vi "_FG_save_hth_v6.vi"(0 "Énum":T1, 1 "array 1":dbl[](array[numeric]), 3 "array 2":dbl[](array[numeric]), 4 "array 3":dbl[](array[numeric]), 5 "error in":errorcluster, 6 "antet_files":string, 7 "write to raw data ?":bool, 8 "add EOL at end ?":bool, 9 "text before data":string, 11 "text":string, 12 "cluster of arrays":cluster{dbl, dbl}[](array[cluster]), 13 "format":string="%12.9g") -> (19 "error out":errorcluster)   [LabVIEW 2017]
uses:
  controls/save_data_hth_v8.ctl
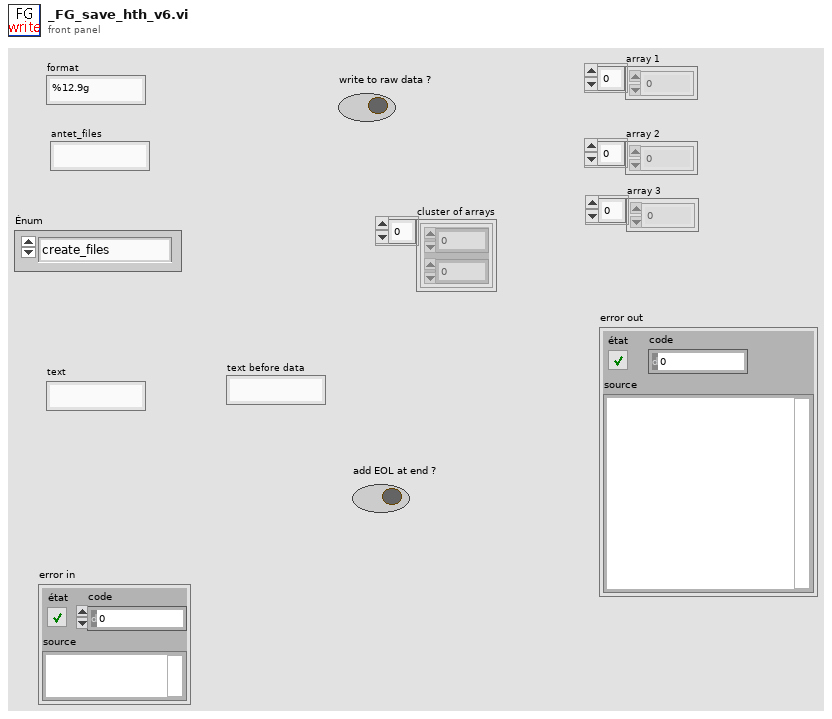
[diagram p1: front panel]
types:
  T1 = typedef "save_data_hth_v8.ctl" = enum16{"create_files", "write_text", "write_array", "w_array_inline", "write_arrays_cluster", "write_eol", "write_time", "close_file"}
  T2 = enum16{"open", "replace", "create", "open or create", "replace or create", "replace or create with confirmation"}
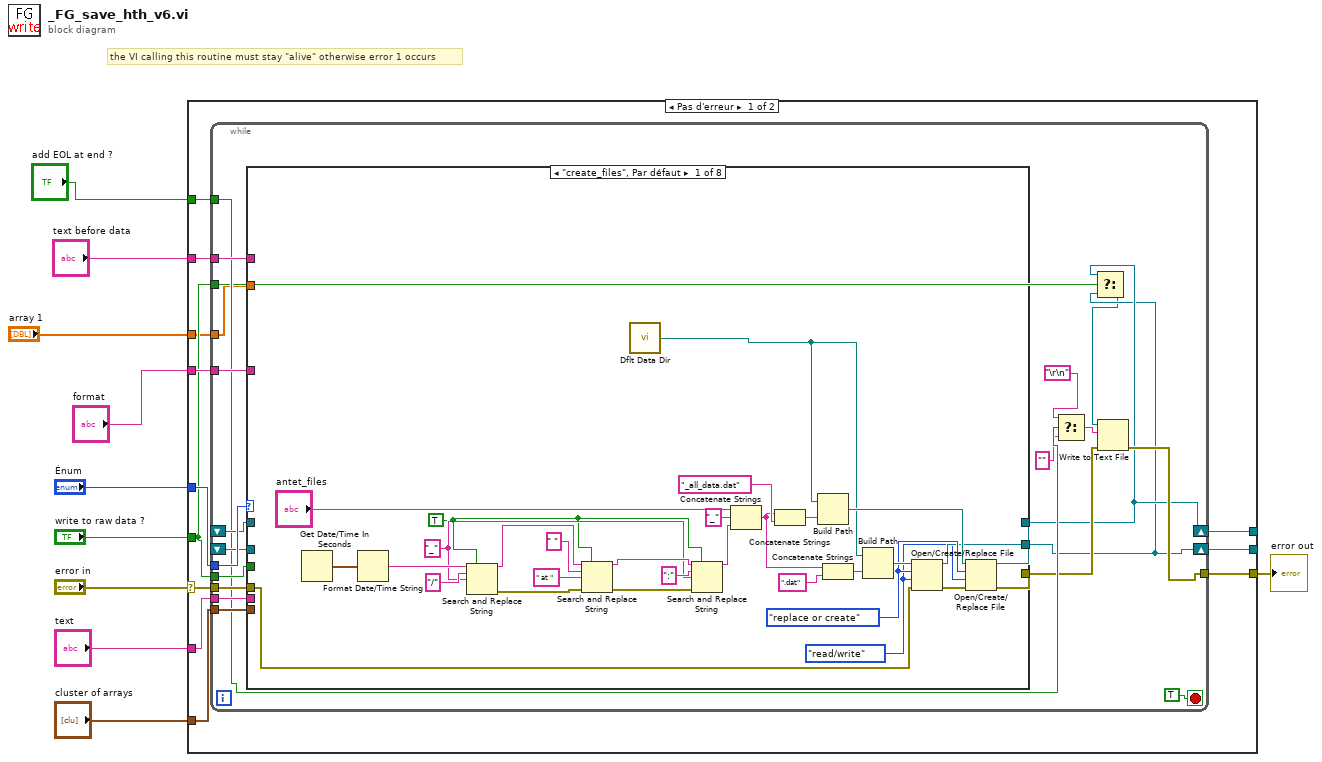
[diagram p0: block diagram]
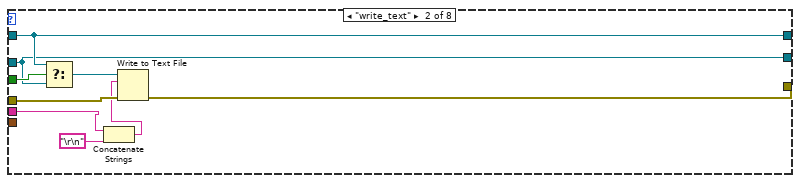
[diagram p2: hidden frame]
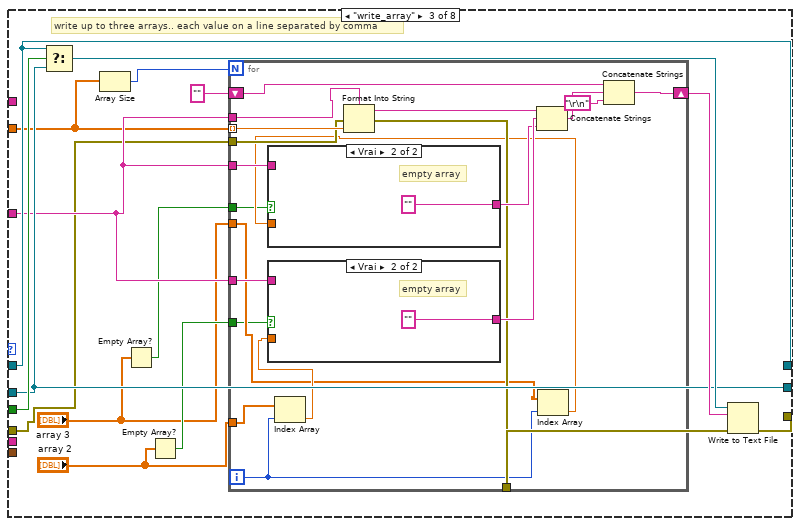
[diagram p3: hidden frame]
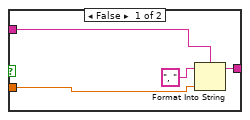
[diagram p4: hidden frame]
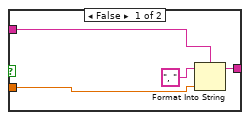
[diagram p5: hidden frame]
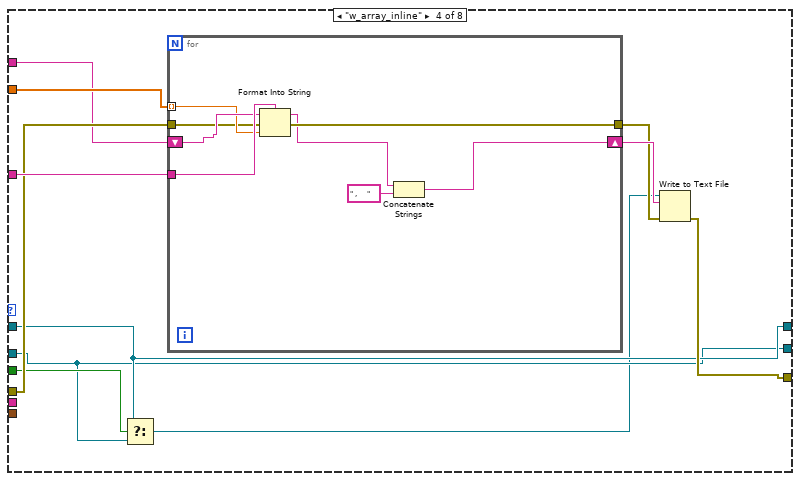
[diagram p6: hidden frame]
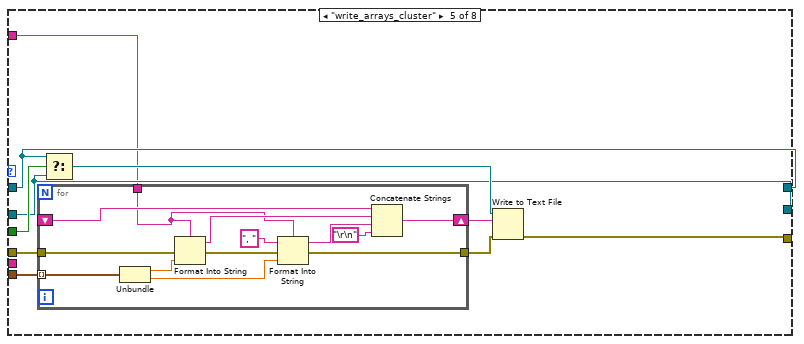
[diagram p7: hidden frame]
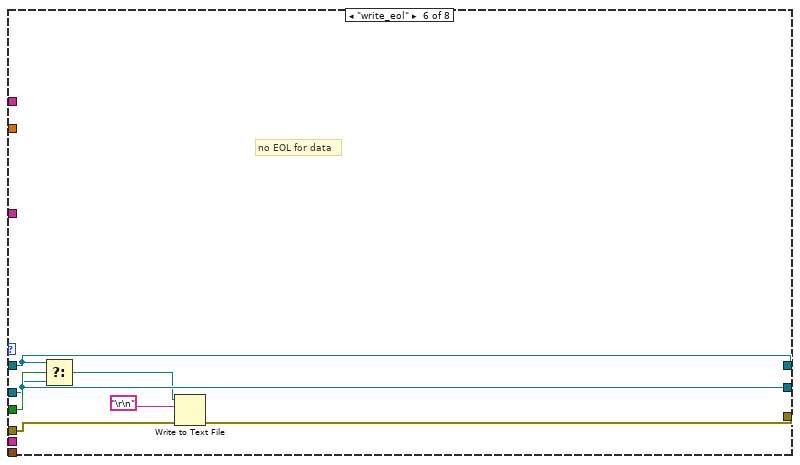
[diagram p8: hidden frame]
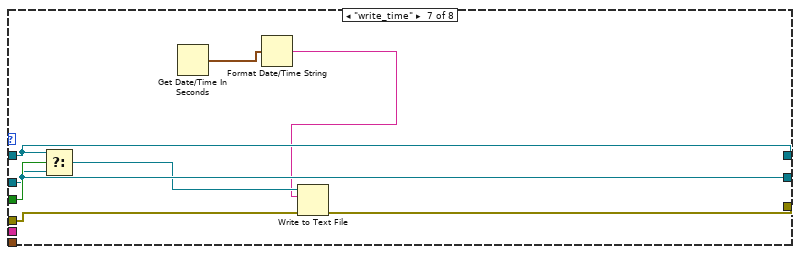
[diagram p9: hidden frame]
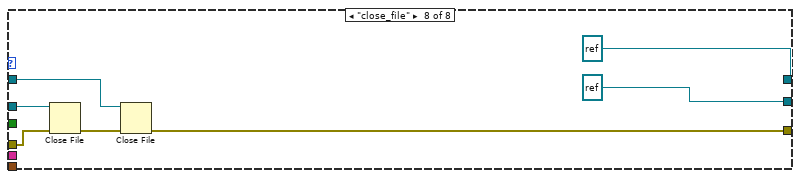
[diagram p10: hidden frame]
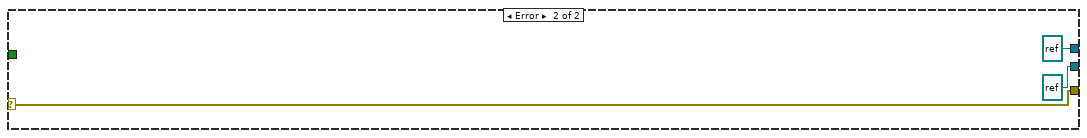
[diagram p11: hidden frame]
diagram:
  # "the VI calling this routine must stay \"alive\" otherwise error 1 occurs"
  n1 = case shown="Pas d'erreur" "error in" {
    selector: "error in" -> [w21 w193]
    tunnel: "Énum" -> [w22 _]
    tunnel: [w20 refnum<file> refnum ("refnum out")] -> _
    tunnel: [w19 refnum<file> refnum ("refnum out")] -> _
    tunnel: [w18 w193] -> w8
    tunnel: "write to raw data ?" -> [w12 _]
    tunnel: "cluster of arrays" -> [w17 _]
    tunnel: "text" -> [w16 _]
    tunnel: "format" -> [w15 _]
    tunnel: "text before data" -> [w14 _]
    tunnel: "add EOL at end ?" -> [w13 _]
    tunnel: "array 1" -> [w11 _]
    frame No Error {
      n2 = while {
        tunnel: w22 -> [w42]
        tunnel: w21 -> [w41]
        shift-right: [w26] -> w20
        shift-left: _ -> [w38]
        shift-right: [w25] -> w19
        shift-left: _ -> [w39]
        tunnel: [w28] -> w18
        tunnel: w12 -> [w40]
        tunnel: w17 -> [w37]
        tunnel: w16 -> [w36]
        tunnel: w15 -> [w35]
        tunnel: w14 -> [w34]
        tunnel: w13 -> [w33]
        tunnel: w12 -> [w27]
        tunnel: w11 -> [w23]
        stop <- TRUE stop-if-true
        n3 = case shown="\"create_files\", Par défaut" w42 {
          tunnel: w41 -> [w58 w82 w90 w137 w149 w172 w180 w191]
          tunnel: [w54 w79 w93 w132 w152 w175 w183 refnum<file> refnum ("refnum out")] -> w26
          tunnel: [w52 w78 w92 w131 w153 w176 w184 refnum<file> refnum ("refnum out")] -> w25
          tunnel: [w50 w81 w94 w134 w151 w173 w181 w188] -> w29
          tunnel: w40 -> [_ w80 w96 w133 w155 w177 w185 _]
          tunnel: w39 -> [_ w78 w92 w131 w153 w176 w184 w192]
          tunnel: w38 -> [_ w79 w93 w132 w152 w175 w183 w189]
          tunnel: w37 -> [_ _ _ _ w157 _ _ _]
          tunnel: w36 -> [_ w75 _ _ _ _ _ _]
          tunnel: w35 -> [_ _ w91 w138 w148 _ _ _]
          tunnel: w34 -> [_ _ _ w129 _ _ _ _]
          tunnel: w23 -> [_ _ w83 w139 _ _ _ _]
          frame "create_files", Default {
            w47 = enum16{"read/write", "read-only", "write-only"}."read/write" ("accès (0 : read/write)")
            w53 = T2."replace or create" ("opération (0 : open)")
            w62 = TRUE ("tout remplacer ? (F)")
            w64 = "_" ("chaîne de remplacement (\"\")")
            n4 = Get Date/Time In Seconds() -> (seconds since 1Jan1904=w73:timestamp)
            n5 = Format Date/Time String(seconds (now)=w73) -> (date/time string=w72:string)  [unwired: 2 in]
            n6 = Search and Replace String(replace all?=w62, input string=w72, search string="/" ("chaîne recherchée"), replace string=w64) -> (result string=w70:string, error out=w63:errorcluster)  [unwired: 4 in, 2 out]
            n7 = Search and Replace String(replace all?=w62, input string=w70, search string=" " ("chaîne recherchée"), replace string=" at " ("chaîne de remplacement (\"\")"), error in=w63) -> (result string=w66:string, error out=w67:errorcluster)  [unwired: 3 in, 2 out]
            n8 = call <vilib>:"Dflt Data Dir.vi"() -> ("App:Default Data Directory"=w44:path)
            n9 = Search and Replace String(replace all?=w62, input string=w66, search string=":" ("chaîne recherchée"), replace string=w64, error in=w67) -> (result string=w46:string)  [unwired: 3 in, 3 out]
            n10 = Concatenate Strings("antet_files", "_" ("chaîne"), w46) -> (w48:string)
            n11 = Concatenate Strings(w48, "_all_data.dat" ("chaîne")) -> (w56:string)
            n12 = Build Path(base path=w44, name or relative path=w56) -> (appended path=w55:path)
            n13 = Concatenate Strings(w48, ".dat" ("chaîne")) -> (w59:string)
            n14 = Build Path(base path=w44, name or relative path=w59) -> (appended path=w61:path)
            n15 = Open/Create/Replace File(file path (use dialog)=w61, error in=w58, operation (0:open)=w53, access (0:read/write)=w47) -> (refnum out=w52:refnum<file>, error out=w51:errorcluster)  [unwired: 2 in, 1 out]
            n16 = Open/Create/Replace File(file path (use dialog)=w55, error in=w51, operation (0:open)=w53, access (0:read/write)=w47) -> (refnum out=w54:refnum<file>, error out=w50:errorcluster)  [unwired: 2 in, 1 out]
          }
          frame "write_text" {
            n17 = Select(t=w79, s=w80, f=w78) -> (s? t:f=w77:refnum<file>)
            n18 = Concatenate Strings(w75, "\r\n") -> (w74:string)
            n19 = Write to Text File(file (use dialog)=w77, text=w74, error in=w82) -> (error out=w81:errorcluster)  [unwired: 1 in, 2 out]
          }
          frame "write_array" {
            # "write up to three arrays.. each value on a line separated by comma"
            n20 = Select(t=w93, s=w96, f=w92) -> (s? t:f=w95:refnum<file>)
            n21 = Array Size(array=w83) -> (size(s)=w88:i32)
            n22 = Empty Array?(array="array 3") -> (empty?=w84:bool)
            n23 = Empty Array?(array="array 2") -> (empty?=w86:bool)
            n24 = for {
              N: w88 -> [_]
              tunnel: w83 -> [w118] mode=indexing
              shift-right: [w116] -> w97
              shift-left: "" -> [w117]
              tunnel: "array 2" -> [w104]
              tunnel: "array 3" -> [w103]
              tunnel: w91 -> [w110]
              tunnel: w91 -> [w109]
              tunnel: w91 -> [w108]
              tunnel: w90 -> [w107]
              tunnel: [w106] -> w89
              tunnel: w86 -> [w100]
              tunnel: w84 -> [w99]
              i -> [w102]
              n25 = Index Array(array=w104, index=w102) -> (element=w105:dbl)
              n26 = case shown="Vrai" w100 {
                tunnel: w105 -> [w127 _]
                tunnel: [w126 ""] -> w114
                tunnel: w108 -> [w124 _]
                frame False {
                  n27 = Format Into String(format string=w124, initial string=", " ("chaîne initiale"), w127) -> (resulting string=w126:string)  [unwired: 1 in, 1 out]
                }
                frame True {
                  # "empty array"
                }
              }
              n28 = Format Into String(format string=w110, error in=w107, w118) -> (resulting string=w115:string, error out=w106:errorcluster)  [unwired: 1 in]
              n29 = Index Array(array=w103, index=w102) -> (element=w101:dbl)
              n30 = case shown="Vrai" w99 {
                tunnel: [w120 ""] -> w113
                tunnel: w101 -> [w122 _]
                tunnel: w109 -> [w119 _]
                frame False {
                  n31 = Format Into String(format string=w119, initial string=", " ("chaîne"), w122) -> (resulting string=w120:string)  [unwired: 1 in, 1 out]
                }
                frame True {
                  # "empty array"
                }
              }
              n32 = Concatenate Strings(w115, w114, w113) -> (w112:string)
              n33 = Concatenate Strings(w117, w112, "\r\n") -> (w116:string)
            }
            n34 = Write to Text File(file (use dialog)=w95, text=w97, error in=w89) -> (error out=w94:errorcluster)  [unwired: 1 in, 2 out]
          }
          frame "w_array_inline" {
            n35 = Select(t=w132, s=w133, f=w131) -> (s? t:f=w130:refnum<file>)
            n36 = for {
              tunnel: w139 -> [w145] mode=indexing
              tunnel: w138 -> [w147]
              shift-right: [w140] -> w136
              shift-left: w129 -> [w146]
              tunnel: w137 -> [w144]
              tunnel: [w143] -> w135
              n37 = Format Into String(format string=w147, initial string=w146, error in=w144, w145) -> (resulting string=w141:string, error out=w143:errorcluster)
              n38 = Concatenate Strings(w141, " ,     " ("chaîne")) -> (w140:string)
            }
            n39 = Write to Text File(file (use dialog)=w130, text=w136, error in=w135) -> (error out=w134:errorcluster)  [unwired: 1 in, 2 out]
          }
          frame "write_arrays_cluster" {
            n40 = for {
              tunnel: w157 -> [w170] mode=indexing
              shift-right: [w164] -> w156
              shift-left: _ -> [w163]
              tunnel: [w161] -> w150
              tunnel: w149 -> [w159]
              tunnel: w148 -> [w158]
              n41 = Unbundle(w170) -> (w169:dbl, w168:dbl)
              n42 = Format Into String(format string=w158, error in=w159, w169) -> (resulting string=w166:string, error out=w160:errorcluster)  [unwired: 1 in]
              n43 = Format Into String(format string=w158, initial string=", " ("chaîne initiale"), error in=w160, w168) -> (resulting string=w165:string, error out=w161:errorcluster)
              n44 = Concatenate Strings(w163, w166, w165, "\r\n") -> (w164:string)
            }
            n45 = Select(t=w152, s=w155, f=w153) -> (s? t:f=w154:refnum<file>)
            n46 = Write to Text File(file (use dialog)=w154, text=w156, error in=w150) -> (error out=w151:errorcluster)  [unwired: 1 in, 2 out]
          }
          frame "write_eol" {
            # "no EOL for data"
            n47 = Select(t=w175, s=w177, f=w176) -> (s? t:f=w174:refnum<file>)
            n48 = Write to Text File(file (use dialog)=w174, text="\r\n", error in=w172) -> (error out=w173:errorcluster)  [unwired: 1 in, 2 out]
          }
          frame "write_time" {
            n49 = Select(t=w183, s=w185, f=w184) -> (s? t:f=w182:refnum<file>)
            n50 = Get Date/Time In Seconds() -> (seconds since 1Jan1904=w179:timestamp)
            n51 = Format Date/Time String(seconds (now)=w179) -> (date/time string=w178:string)  [unwired: 2 in]
            n52 = Write to Text File(file (use dialog)=w182, text=w178, error in=w180) -> (error out=w181:errorcluster)  [unwired: 1 in, 2 out]
          }
          frame "close_file" {
            n53 = Close File(refnum=w192, error in=w191) -> (error out=w190:errorcluster)  [unwired: 1 out]
            n54 = Close File(refnum=w189, error in=w190) -> (error out=w188:errorcluster)  [unwired: 1 out]
          }
        }
        n55 = Select(t="\r\n", s=w33, f="" ("cas faux")) -> (s? t:f=w30:string)
        n56 = Select(t=w26, s=w27, f=w25) -> (s? t:f=w24:refnum<file>)
        n57 = Write to Text File(file (use dialog)=w24, text=w30, error in=w29) -> (error out=w28:errorcluster)  [unwired: 1 in, 2 out]
      }
    }
    frame Error {
    }
  }
  "error out" <- w8
